vi "LJstreamUD data file write.vi"(0 "Current Data File In":path, 1 "Write To File":bool, 3 "Data File Prefix":string="data", 5 "Voltages":dbl[][](array[numeric]) format="%.3f", 6 "Time":dbl format="%.2f", 9 "Scaled Data":dbl[][](array[numeric]) format="%.3f", 11 "max file size (bytes)":i32=100000000, 12 "Channel Config":T1={"# Channels"=4, "+Ch"=["0", "1", "2", "3", "4", "5", "6", "7"], "-Ch (U3)"=["31", "31", "31", "31", "31", "31", "31", "31"], "Ranges (UE9)"=[0, 0, 0, 0, 0, 0, 0, 0], "Scaling Equation"=["y=v0", "y=v1", "y=v2", "y=v3", "y=v4", "y=v5", "y=v6", "y=v7"]} {"Ranges (UE9)" items=["LJ_rgBIP5V", "LJ_rgUNI5V", "LJ_rgUNI2P5V", "LJ_rgUNI1P25V", "LJ_rgUNIP625V"]}, 13 "Disable Scaling":bool, 14 "Scan Rate":dbl=50.0 format="%.2f", 15 "Starting #":u32) -> (4 "Current Data File Out":path, 10 "Data File #":u32)   [LabVIEW 2020]
uses:
  LJstreamUD globals.vi
panel:
  out "ms":u32
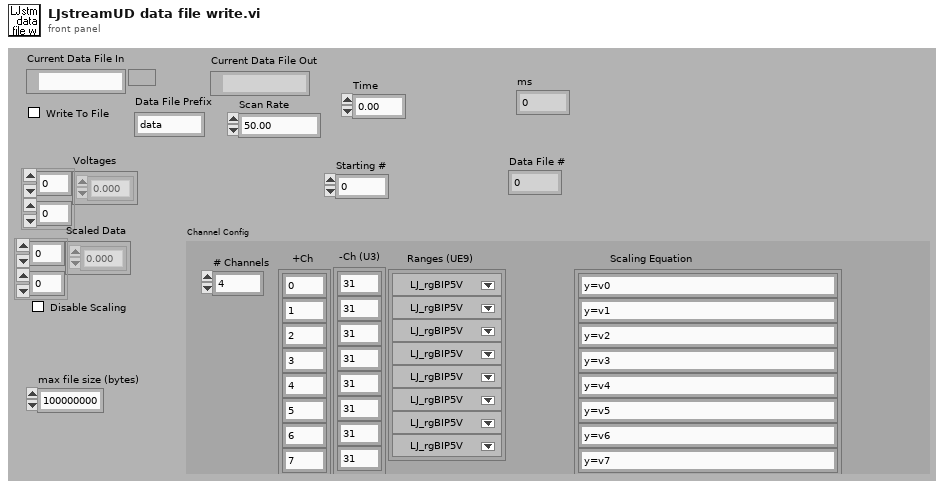
[diagram p1: front panel]
types:
  T1 = cluster{"# Channels":i32, "+Ch":string[], "-Ch (U3)":string[], "Ranges (UE9)":u16[], "Scaling Equation":string[]}
  T2 = enum16{"open", "open or create", "create or replace", "create", "open (read only)"}
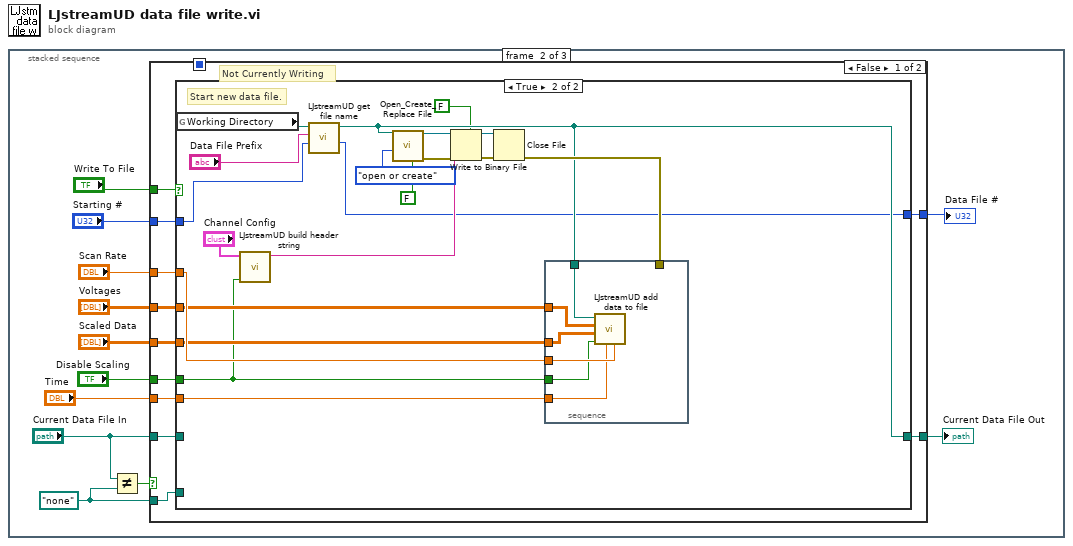
[diagram p0: block diagram]
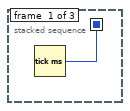
[diagram p2: hidden frame]
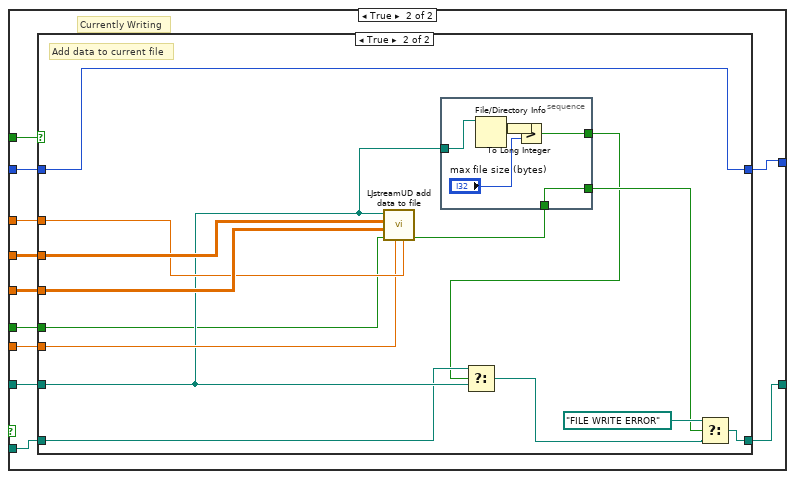
[diagram p4: hidden frame]
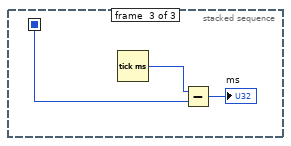
[diagram p6: hidden frame]
diagram:
  n1 = stacked-sequence {
    seq-local: [w1 _ _] -> [_ _ w87]
    frame #0 {
      n2 = Tick Count (ms)() -> (millisecond timer value=w1:u32)
    }
    frame #1 {
      w9 = path "none" ("y")
      n3 = Not Equal?(x="Current Data File In", y=w9) -> (x != y?=w13:bool)
      n4 = case shown="False" w13 {
        tunnel: "Current Data File In" -> [w24 w63]
        tunnel: "Write To File" -> [w22 w62]
        tunnel: [w23 w60] -> w10
        tunnel: w9 -> [w21 w61]
        tunnel: "Voltages" -> [w18 w59]
        tunnel: "Scaled Data" -> [w17 w58]
        tunnel: "Scan Rate" -> [w20 w57]
        tunnel: "Time" -> [w19 w56]
        tunnel: "Starting #" -> [w16 w55]
        tunnel: [w15 w54] -> w3
        tunnel: "Disable Scaling" -> [w14 w53]
        frame False {
          # "Not Currently Writing"
          n5 = case shown="True" w22 {
            tunnel: w24 -> [_ _]
            tunnel: [w26 w37] -> w23
            tunnel: w21 -> [w26 _]
            tunnel: w20 -> [_ w36]
            tunnel: w19 -> [_ w35]
            tunnel: w18 -> [_ w34]
            tunnel: w17 -> [_ w33]
            tunnel: w16 -> [w25 w30]
            tunnel: [w25 w29] -> w15
            tunnel: w14 -> [_ w28]
            frame False {
              # "Do nothing"
            }
            frame True {
              # "Start new data file."
              n6 = global read "LJstreamUD globals.vi" "Working Directory"() -> (w32:path)
              n7 = call "LJstreamUD build header string.vi"("Disable Scaling"=w28, "Channel Config"="Channel Config") -> ("Header String"=w39:string)  [unwired: 9 in]
              n8 = call "LJstreamUD get file name.vi"("Starting #"=w30, "Data File Prefix"="Data File Prefix", "Working Directory"=w32) -> ("Data File #"=w29:u32, "Data File Path"=w37:path)  [unwired: 7 in]
              n9 = call <vilib>:"Open_Create_Replace File.vi"("advisory dialog? (display:T)"=FALSE, "function (open:0)"=T2."open or create", "file path"=w37) -> ("error out"=w43:errorcluster, "refnum"=w42:refnum<file>)  [unwired: 5 in, 2 out]
              n10 = Write to Binary File(file (use dialog)=w42, data=w39, error in=w43, 5:FALSE ("prepend array or string size? (T)")) -> (refnum out=w40:refnum<file>, error out=w41:errorcluster)  [unwired: 2 in, 1 out]
              n11 = Close File(refnum=w40, error in=w41) -> (error out=w38:errorcluster)  [unwired: 1 out]
              n12 = stacked-sequence {
                tunnel: w38 -> [_]
                tunnel: w37 -> [w52]
                tunnel: w36 -> [w51]
                tunnel: w35 -> [w50]
                tunnel: w34 -> [w49]
                tunnel: w33 -> [w48]
                tunnel: w28 -> [w47]
                frame #0 {
                  n13 = call "LJstreamUD add data to file.vi"("Scan Rate"=w51, "Time"=w50, "Disable Scaling"=w47, "Scaled Data"=w48, "Voltages"=w49, "file path"=w52) -> ()  [unwired: 5 in, 1 out]
                }
              }
            }
          }
        }
        frame True {
          # "Currently Writing"
          n14 = case shown="True" w62 {
            tunnel: w63 -> [_ w71]
            tunnel: [w65 w72] -> w60
            tunnel: w61 -> [w65 w69]
            tunnel: w59 -> [_ w78]
            tunnel: w58 -> [_ w77]
            tunnel: w57 -> [_ w76]
            tunnel: w56 -> [_ w75]
            tunnel: w55 -> [w64 w67]
            tunnel: [w64 w67] -> w54
            tunnel: w53 -> [_ w66]
            frame False {
              # "Stop writing to current data file."
            }
            frame True {
              # "Add data to current file"
              n15 = call "LJstreamUD add data to file.vi"("Scan Rate"=w76, "Time"=w75, "Disable Scaling"=w66, "Scaled Data"=w77, "Voltages"=w78, "file path"=w71) -> ("error"=w74:bool)  [unwired: 5 in]
              n16 = stacked-sequence {
                tunnel: w74 -> [w85]
                tunnel: [w85] -> w73
                tunnel: w71 -> [w84]
                tunnel: [w82] -> w68
                frame #0 {
                  n17 = File/Directory Info(path=w84) -> (size=w80:i64)  [unwired: 1 in, 6 out]
                  n18 = To Long Integer(number=w80) -> (32bit integer=w83:i32)
                  n19 = Greater?(x=w83, y="max file size (bytes)") -> (0:w82:bool)
                }
              }
              n20 = Select(t=w69, s=w68, f=w71) -> (s? t:f=w70:path)
              n21 = Select(t=path "FILE WRITE ERROR", s=w73, f=w70) -> (s? t:f=w72:path)
            }
          }
        }
      }
      "Current Data File Out" <- w10
      "Data File #" <- w3
    }
    frame #2 {
      n22 = Tick Count (ms)() -> (millisecond timer value=w88:u32)
      n23 = Subtract(x=w88, y=w87) -> (x-y=→"ms":u32)
    }
  }
